vi "Spartan Version.vi"() -> ()   [LabVIEW 2011]
uses:
  Summitek EXT/Miscellaneous/OGAB Version.ctl
panel:
  out "Pause TDMS Organization":bool
  out "Debug":bool
  out "Web Server Path":path
  out "Web Server Port":u16
  out "STOPPED":bool
  in  "Version":T1={"Version"="6.3", "Build Number"=12, "Build Date/Time"=3440694548.419435} {"Build Date/Time" format="%<%X\n%x>T"}
  # "Note: The version\nglobal is set during\nbuild.  Don't change\nor rename this variable"
  # "The Web Server Path and Web Server Port\ncontrols are necessary for client interaction.\nThese values cannot be read remotely, so\nwe need to do a global call to get these values\non the client side.  DO NOT DELETE!!!"
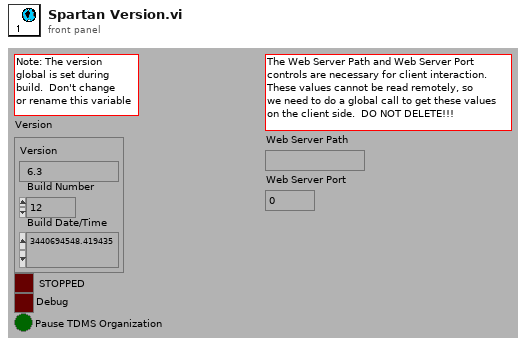
[diagram p1: front panel]
types:
  T1 = typedef "OGAB Version.ctl" = cluster{"Version":string, "Build Number":u32, "Build Date/Time":dbl}
diagram:
